vi "ReadDefaultSchedules.vi"(10 "File Name":string) -> (0 "Times Called":dbl, 1 "Scheduler":T1(array[cluster]), 2 "File Exists":bool)   [LabVIEW 2018]
panel:
  out "Numeric":dbl
  out "File Path":path
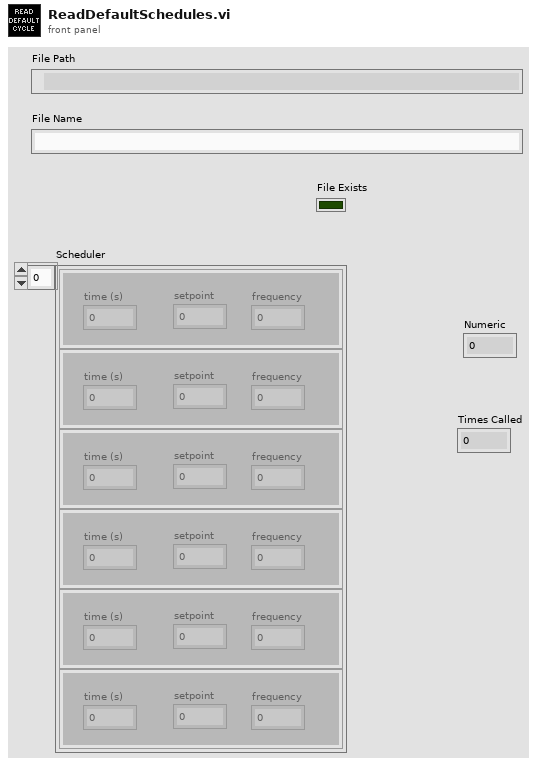
[diagram p1: front panel]
types:
  T1 = cluster{"time (s)":dbl, "setpoint ":dbl, "frequency":dbl}[]
  T2 = cluster{"[0]":dbl, "[1]":dbl, "[2]":dbl, "[3]":dbl, "[4]":dbl, "[5]":dbl, "[6]":dbl, "[7]":dbl, "[8]":dbl}
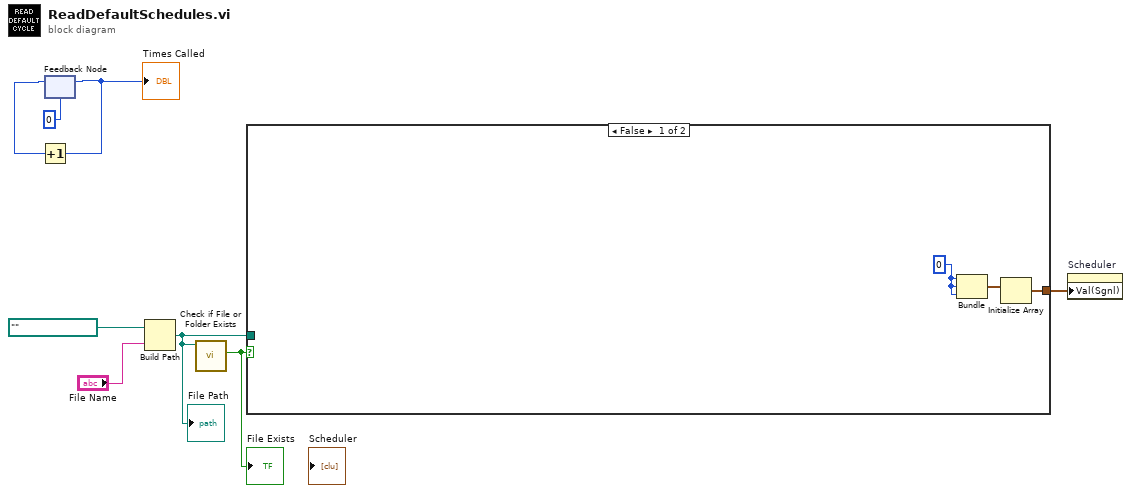
[diagram p0: block diagram]
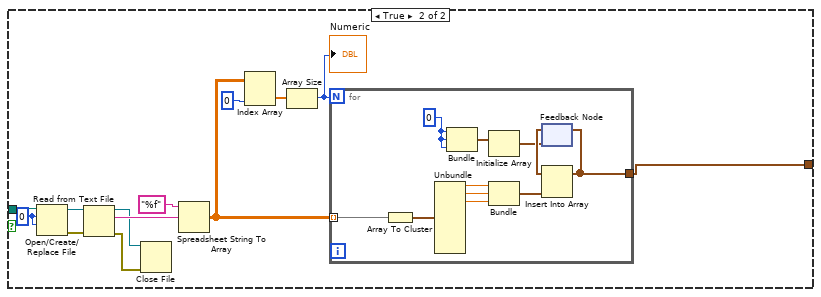
[diagram p2: hidden frame]
diagram:
  n1 = feedback #1(0) -> (w3:i32)
  n2 = Increment(x=w3) -> (x+1=w2:i32)
  "Times Called" <- w2
  n3 = feedback-in #1(w2) -> ()
  n4 = Build Path(base path=path "", name or relative path="File Name") -> (appended path=w6:path)
  "File Path" <- w6
  n5 = call <vilib>:"Check if File or Folder Exists.vi"("path"=w6) -> ("file or folder exists?"=w7:bool)  [unwired: 8 in, 2 out]
  "File Exists" <- w7
  n6 = case shown="False" w7 {
    tunnel: w6 -> [_ w13]
    tunnel: [w9 w18] -> w5
    frame False {
      w11 = 0
      n7 = Bundle(w11, w11, w11) -> (w10:cluster{i32, i32, i32})  [unwired: 1 in]
      n8 = Initialize Array(w10) -> (w9:cluster{i32, i32, i32}[])  [unwired: 1 in]
    }
    frame True {
      w12 = 0
      n9 = Open/Create/Replace File(file path (use dialog)=w13, operation (0:open)=w12, access (0:read/write)=w12) -> (refnum out=w14:refnum<file>, error out=w16:errorcluster)  [unwired: 3 in, 1 out]
      n10 = Read from Text File(file (use dialog)=w14, error in=w16) -> (refnum out=w17:refnum<file>, text=w24:string, error out=w15:errorcluster)  [unwired: 2 in, 1 out]
      n11 = Close File(refnum=w17, error in=w15) -> ()  [unwired: 2 out]
      n12 = Spreadsheet String To Array(format string="%f", spreadsheet string=w24) -> (array=w22:dbl[][])  [unwired: 2 in]
      n13 = Index Array(array=w22, index (col)=0) -> (element=w21:dbl[])  [unwired: 1 in]
      n14 = Array Size(array=w21) -> (size(s)=w19:i32)
      "Numeric" <- w19
      n15 = for {
        N: w19 -> [_]
        tunnel: w22 -> [w35] mode=indexing
        tunnel: [w28] -> w18
        w26 = 0
        n16 = Array To Cluster(array=w35) -> (cluster=w34:T2)
        n17 = Unbundle(w34) -> ("[0]"=w33:dbl, "[1]"=w32:dbl, "[2]"=w31:dbl)  [unwired: 6 out]
        n18 = Bundle(w26, w26, w26) -> (w27:cluster{i32, i32, i32})  [unwired: 1 in]
        n19 = Initialize Array(w27) -> (w25:cluster{i32, i32, i32}[])  [unwired: 1 in]
        n20 = Bundle("[0]"=w33, "[1]"=w32, "[2]"=w31) -> (w30:cluster{"[0]":dbl, "[1]":dbl, "[2]":dbl})  [unwired: 1 in]
        n21 = feedback #2(w25) -> (w29:cluster{i32, i32, i32}[])
        n22 = Insert Into Array(array=w29, new element=w30) -> (w28:cluster{i32, i32, i32}[])  [unwired: 1 in]
        n23 = feedback-in #2(w28) -> ()
      }
    }
  }
  n24 = property on="Scheduler" class="Arr (strict)"("Val(Sgnl)"=w5) -> ()  [unwired: 2 in, 2 out]
